vi "Apply Module Selection.vi"(8 "error in (no error)":errorcluster, 9 "Module Type":T1, 10 "Slot # in":i32, 11 "Base Topology Variant in":variant) -> (0 "error out":errorcluster, 3 "Base Topology Variant out":variant)   [LabVIEW 2017]
uses:
  Slot Module Selection.ctl
  Module Type.ctl
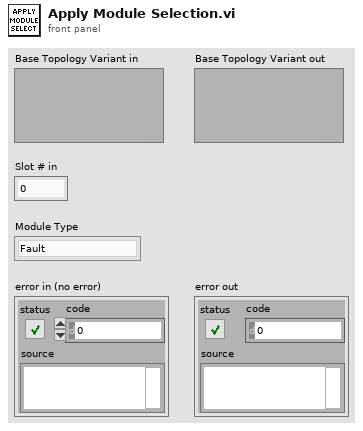
[diagram p1: front panel]
types:
  T1 = typedef "Slot Module Selection.ctl" = enum16{"Fault", "Instrument", "Empty"}
  T2 = typedef "Module Type.ctl" = enum16{"Fault", "Instrument"}
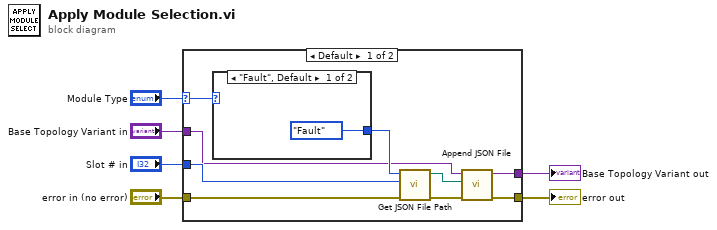
[diagram p0: block diagram]
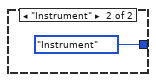
[diagram p2: hidden frame]
diagram:
  n1 = case shown="Default" "Module Type" {
    selector: "Module Type" -> [w7 _]
    tunnel: "Slot # in" -> [w14 _]
    tunnel: [w11 w19] -> w5
    tunnel: "Base Topology Variant in" -> [w10 w19]
    tunnel: "error in (no error)" -> [w9 w18]
    tunnel: [w8 w18] -> w2
    frame Default {
      n2 = case shown="\"Fault\", Default" w7 {
        tunnel: [Module_Type."Fault" ("Slot 1 Module Type") Module_Type."Instrument" ("Slot 1 Module Type")] -> w13
        frame "Fault", Default {
        }
        frame "Instrument" {
        }
      }
      n3 = call "Get JSON File Path.vi"("error in (no error)"=w9, "Slot #"=w14, "Slot 1 Module Type"=w13) -> ("error out"=w12:errorcluster, "appended path"=w15:path)  [unwired: 7 in]
      n4 = call "Append JSON File.vi"("error in (no error)"=w12, "Path"=w15, "Element in"=w10) -> ("error out"=w8:errorcluster, "Base Topology Variant out"=w11:variant)  [unwired: 7 in]
    }
    frame "Empty" {
    }
  }
  "Base Topology Variant out" <- w5
  "error out" <- w2
